vi "Set speed graph Y-range.vi"(8 "error in (no error)":errorcluster, 11 "Speed max/min":cluster{"max value":dbl, "min value":dbl}) -> (0 "error out":errorcluster)   [LabVIEW 2013]
uses:
  Globals/gl_Time series viewer globals.vi
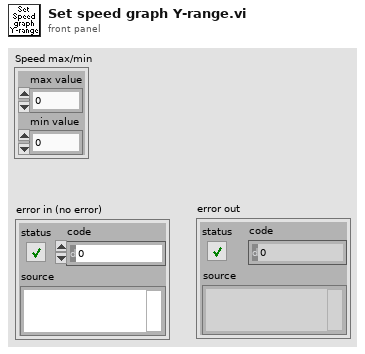
[diagram p1: front panel]
types:
  T1 = typedef "Timelapse viewer refs.ctl" = cluster{"This VI":refnum<vi>, "AVI Mode ind":refnum<vi>, "Play":refnum<vi>, "Stop":refnum<vi>, "Back":refnum<vi>, "Scrollbar":refnum<vi>, "Video length info":refnum<vi>, "Expected speed values":refnum<vi>, "Intensity":refnum<vi>, "Path":refnum<vi>, "Selection sliders":refnum<vi>, "Speed Graph ref":refnum<vi>, "Frame rate set (fps)":refnum<vi>}
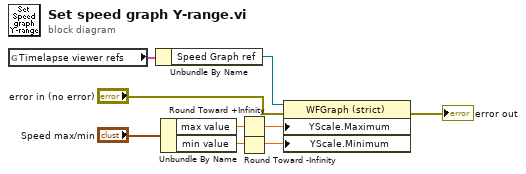
[diagram p0: block diagram]
diagram:
  n1 = global read "gl_Time series viewer globals.vi" "Timelapse viewer refs"() -> (w3:T1)
  n2 = Unbundle By Name(w3) -> ("Speed Graph ref"=w2:refnum<vi>)
  n3 = Unbundle By Name("Speed max/min") -> ("max value"=w8:dbl, "min value"=w7:dbl)
  n4 = Round Toward +Infinity(x=w8) -> (ceil(x): smallest int >= x=w6:dbl)
  n5 = Round Toward -Infinity(1:w7) -> (0:w5:dbl)
  n6 = property on="Property Node" class="WFGraph (strict)"(reference=w2, error in="error in (no error)", "YScale.Maximum"=w6, "YScale.Minimum"=w5) -> (error out=→"error out":errorcluster)  [unwired: 1 out]
